vi "WC_Drive_MotionMagic_DriveMotors.vi"(8 "Error":errorcluster, 11 "RobotDriveDevRef":T1={"DevStatus"={"status"=FALSE, "code"=0, "source"=""}, "Motors[]"=[], "Square Inputs"=FALSE, "Max Output"=1.0}) -> (0 "Error Out":errorcluster, 3 "RobotDriveDevRef Out":T1={"DevStatus"={"status"=FALSE, "code"=0, "source"=""}, "Motors[]"=[], "Square Inputs"=FALSE, "Max Output"=1.0})   [LabVIEW 2017]
doc: "Determines the motor configuration and sends the speed values to the appropriate motors.\n\nThis software is licensed. Open the labview\\readme\\WPI Robotics Library Open Source License.txt file for more information."
uses:
  <vilib>/Rock Robotics/WPI/RobotDrive/WPI_RobotDriveDevRef.ctl
  <vilib>/Rock Robotics/WPI/MotorControl/WPI_MotorControlDeviceRef.ctl
  <vilib>/Rock Robotics/WPI/MotorControl/WPI_MotorControlType.ctl
  <vilib>/Rock Robotics/SystemInterfaces/DIO/FPGA_DIOPWMChannel.ctl
  <vilib>/Rock Robotics/WPI/PWM/WPI_PWMDeadband.ctl
  <vilib>/Rock Robotics/SystemInterfaces/DIO/FPGA_DIOChannel.ctl
  C:/Users/Public/Documents/Cross The Road Electronics/Phoenix-LabVIEW/Motor Controller/Controls/CTRE_Phoenix_MotorControl_ControlMode.ctl
panel:
  in  "Accel":i32
  in  "Cruis v":i32
  in  "targer":dbl
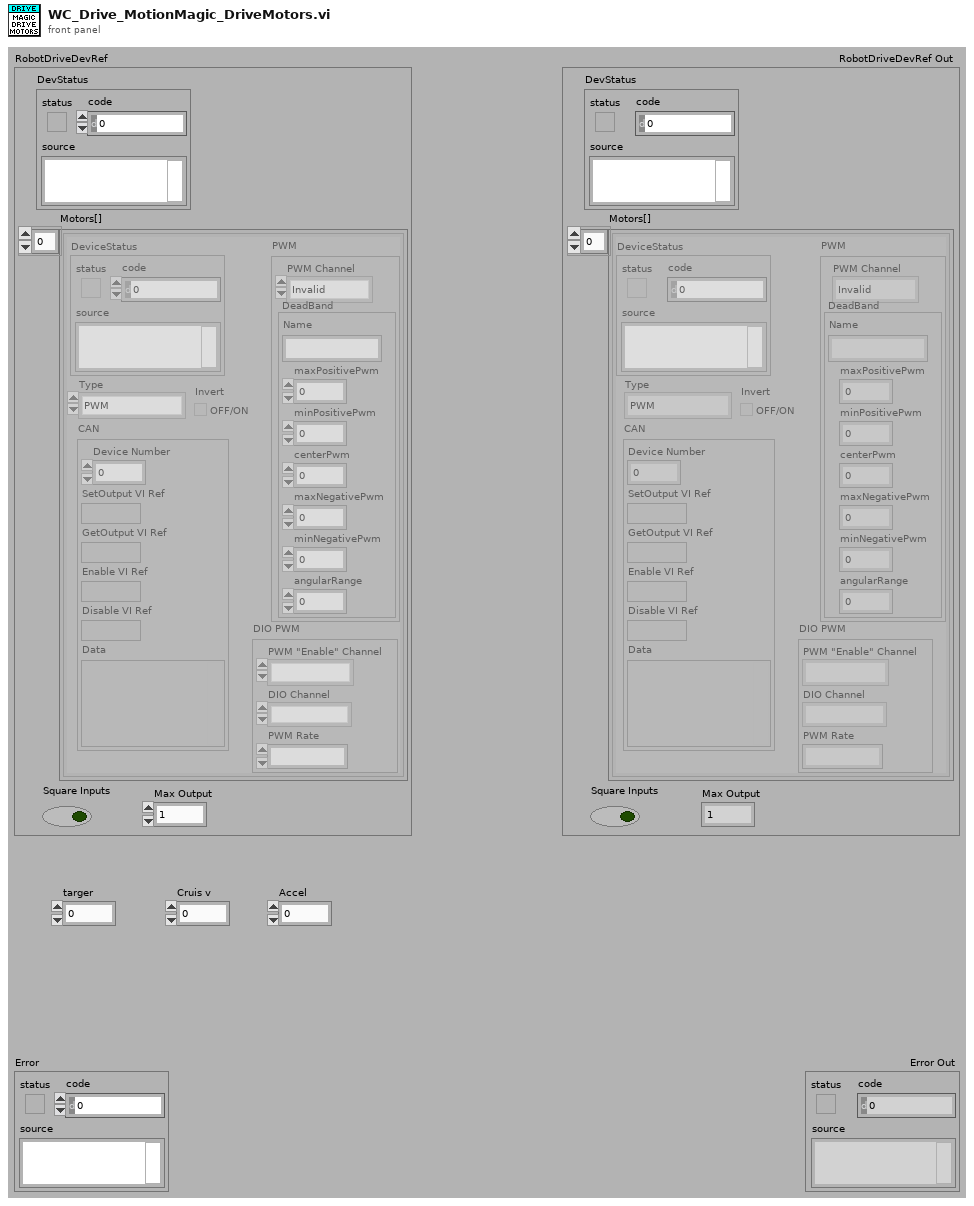
[diagram p1: front panel]
types:
  T1 = typedef "WPI_RobotDriveDevRef.ctl" = cluster{"DevStatus":errorcluster, "Motors[]":T2[], "Square Inputs":bool, "Max Output":dbl}
  T2 = typedef "WPI_MotorControlDeviceRef.ctl" = cluster{"DeviceStatus":errorcluster, "Type":T3, "PWM":cluster{"PWM Channel":T4, "DeadBand":T5}, "CAN":cluster{"Device Number":u8, "SetOutput VI Ref":variant, "GetOutput VI Ref":variant, "Enable VI Ref":variant, "Disable VI Ref":variant, "Data":variant}, "Invert":bool, "DIO PWM":cluster{"PWM \"Enable\" Channel":T4, "DIOChannel":T6, "PWM Rate":dbl}}
  T3 = typedef "WPI_MotorControlType.ctl" = enum16{"PWM", "CAN", "DIO PWM"}
  T4 = typedef "FPGA_DIOPWMChannel.ctl" = enum8{"PWM 0", "PWM 1", "PWM 2", "PWM 3", "PWM 4", "PWM 5", "PWM 6", "PWM 7", "PWM 8", "PWM 9", "PWM MXP 0", "PWM MXP 1", "PWM MXP 2", "PWM MXP 3", "PWM MXP 4", "PWM MXP 5", "PWM MXP 6", "PWM MXP 7", "PWM MXP 8", "PWM MXP 9", "Invalid"}
  T5 = typedef "WPI_PWMDeadband.ctl" = cluster{"Name":string, "maxPositivePwm":i32, "minPositivePwm":i32, "centerPwm":i32, "maxNegativePwm":i32, "minNegativePwm":i32, "angularRange":u16}
  T6 = typedef "FPGA_DIOChannel.ctl" = enum8{"DIO 0", "DIO 1", "DIO 2", "DIO 3", "DIO 4", "DIO 5", "DIO 6", "DIO 7", "DIO 8", "DIO 9", "DIO MXP 0", "DIO MXP 1", "DIO MXP 2", "DIO MXP 3", "DIO MXP 4", "DIO MXP 5", "DIO MXP 6", "DIO MXP 7", "DIO MXP 8", "DIO MXP 9", "DIO MXP 10", "DIO MXP 11", "DIO MXP 12", "DIO MXP 13", "DIO MXP 14", "DIO MXP 15", "SPI Port CS1", "SPI Port CS2", "SPI Port CS3", "SPI Port MISO", "SPI Port MOSI", "Invalid"}
  T7 = typedef "CTRE_Phoenix_MotorControl_ControlMode.ctl" = u16
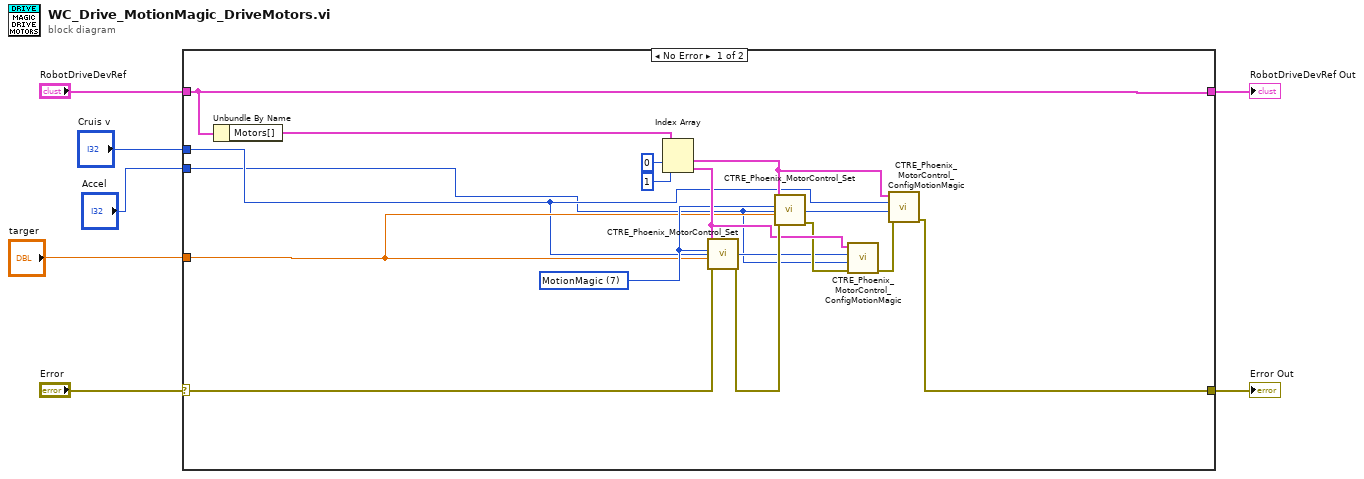
[diagram p0: block diagram]
diagram:
  n1 = case shown="No Error" "Error" {
    selector: "Error" -> [w18 w24]
    tunnel: "RobotDriveDevRef" -> [w19 w23]
    tunnel: [w19 w23] -> w6
    tunnel: [w12 w24] -> w4
    tunnel: "targer" -> [w10 _]
    tunnel: "Cruis v" -> [w9 _]
    tunnel: "Accel" -> [w8 _]
    frame No Error {
      w11 = T7 7 items=["PercentOutput"=0, "Position"=1, "Velocity"=2, "Current"=3, "Follower"=5, "MotionProfile"=6, "MotionMagic"=7, "MotionMagicArc"=8, "MotionProfileArc"=10, "Disabled"=15] ("Control Mode")
      n2 = Unbundle By Name(w19) -> ("Motors[]"=w20:T2[])
      n3 = Index Array(array=w20, index #1=0 ("index"), index #2=1 ("index")) -> (element #1=w15:T2, element #2=w16:T2)
      n4 = call "CTRE_Phoenix_MotorControl_Set.vi"("error in (no error)"=w18, "Output"=w10, "Control Mode"=w11, "PhoenixMotorControlDevRef"=w16) -> ("error out"=w17:errorcluster)  [unwired: 6 in, 1 out]
      n5 = call "CTRE_Phoenix_MotorControl_Set.vi"("error in (no error)"=w17, "Output"=w10, "Control Mode"=w11, "PhoenixMotorControlDevRef"=w15) -> ("error out"=w14:errorcluster)  [unwired: 6 in, 1 out]
      n6 = call "CTRE_Phoenix_MotorControl_ConfigMotionMagic.vi"("error in (no error)"=w14, "Acceleration"=w8, "Cruise Velocity"=w9, "PhoenixMotorControlDevRef"=w16) -> ("error out"=w13:errorcluster)  [unwired: 6 in, 1 out]
      n7 = call "CTRE_Phoenix_MotorControl_ConfigMotionMagic.vi"("error in (no error)"=w13, "Acceleration"=w8, "Cruise Velocity"=w9, "PhoenixMotorControlDevRef"=w15) -> ("error out"=w12:errorcluster)  [unwired: 6 in, 1 out]
    }
    frame Error {
    }
  }
  "RobotDriveDevRef Out" <- w6
  "Error Out" <- w4
